vi "ABB Locked rotor report.vi"(10 "Report in":string) -> (2 "Report out":string, 3 "jpg  path":path)   [LabVIEW 2017]
uses:
  ABB global.vi
panel:
  out "Current Vs. Voltage":T1(graph)
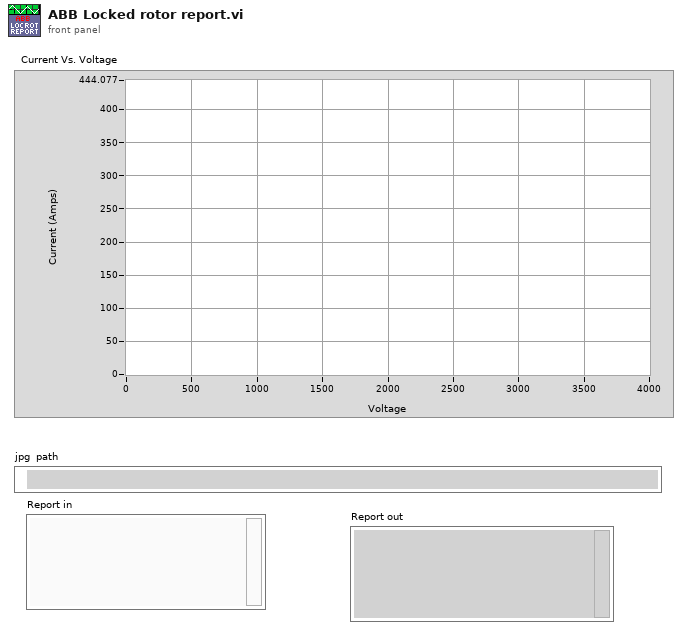
[diagram p1: front panel]
types:
  T1 = cluster{"No load test results":dbl[], "No load test results":dbl[]}
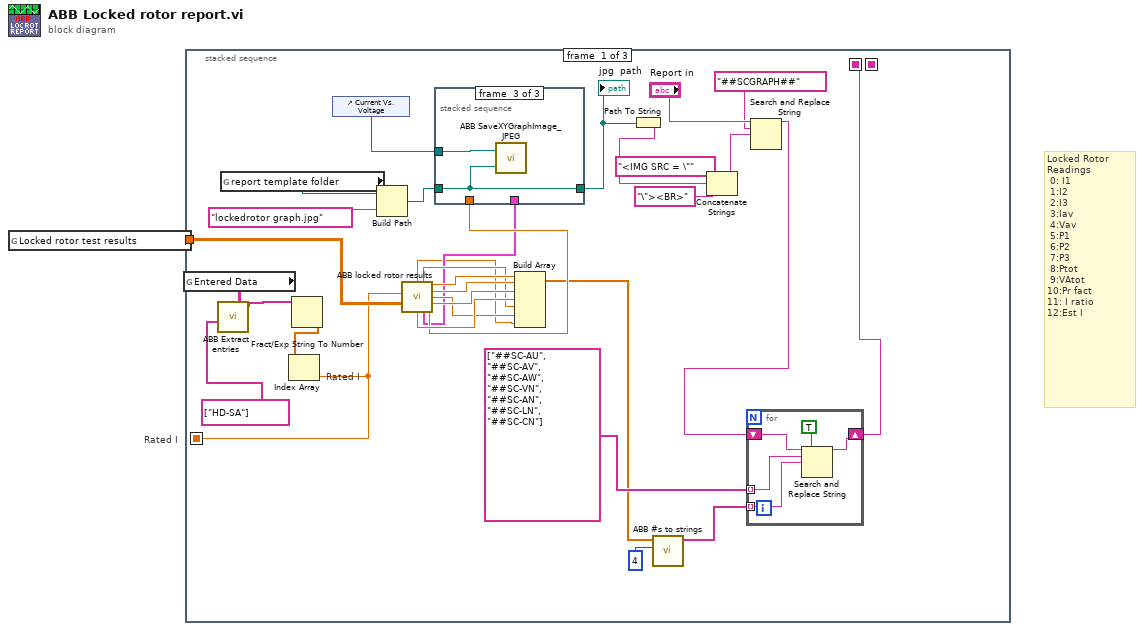
[diagram p0: block diagram]
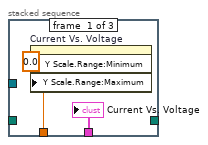
[diagram p2: hidden frame]
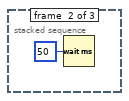
[diagram p3: hidden frame]
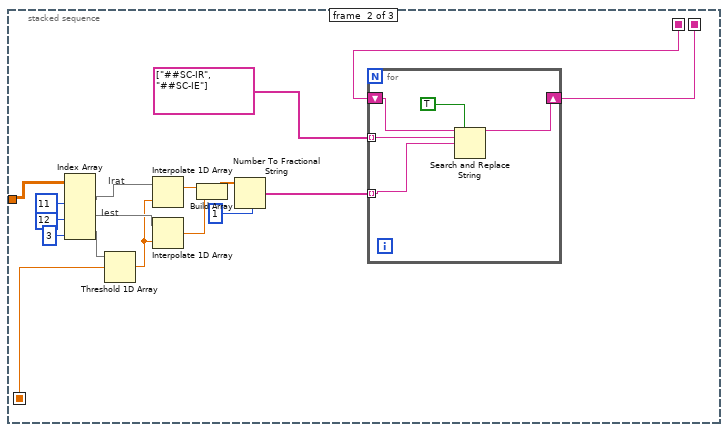
[diagram p4: hidden frame]
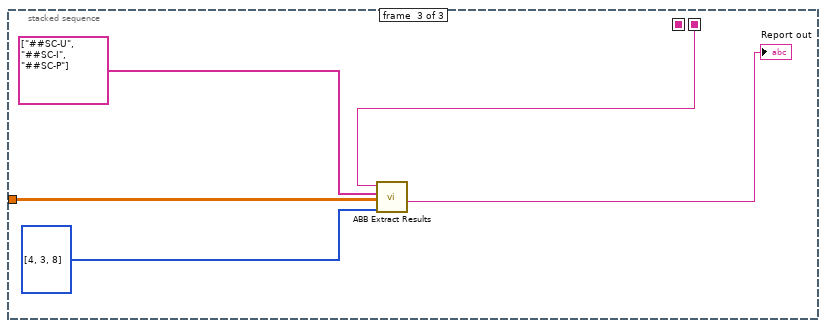
[diagram p5: hidden frame]
diagram:
  # "Rated I"
  # "Locked Rotor\nReadings\n 0: I1\n 1:I2\n 2:I3\n 3:Iav\n 4:Vav\n 5:P1\n 6:P2\n 7:P3\n 8:Ptot\n 9:VAtot\n10:Pr fact\n11: I ratio\n12:Est I"
  n1 = global read "ABB global.vi" "Locked rotor test results"() -> (w1:dbl[][])
  n2 = stacked-sequence {
    seq-local: [w20 _ _] -> [_ w49 _]
    seq-local: [_ w46 _] -> [_ _ w67]
    seq-local: [w3 _ _] -> [_ w45 _]
    tunnel: w1 -> [w15 w50 w71]
    frame #0 {
      # "Rated I"
      n3 = global read "ABB global.vi" "Entered Data"() -> (w23:string[][])
      n4 = call "ABB Extract entries.vi"("Entry IDs"=string[] ["HD-SA"], "Entry table in"=w23) -> ("Selected Entries"=w21:string[])  [unwired: 9 in]
      n5 = global read "ABB global.vi" "report template folder"() -> (w32:path)
      n6 = Fract/Exp String To Number(string=w21) -> (number=w14:dbl[])  [unwired: 3 in, 1 out]
      n7 = Index Array(array=w14) -> (element=w3:dbl)  [unwired: 1 in]
      n8 = control-ref of="Current Vs. Voltage"() -> (w33:refnum<vi>)
      n9 = Build Path(base path=w32, name or relative path="lockedrotor graph.jpg") -> (appended path=w28:path)
      n10 = call "ABB locked rotor results.vi"("Rated Current"=w3, "Locked rotor test results"=w15) -> ("PFr"=w4:dbl, "I AVr"=w9:dbl, "IUr"=w13:dbl, "IVr"=w12:dbl, "PWr"=w8:dbl, "IWr"=w11:dbl, "V AVr"=w10:dbl, "Graph"=w6:T1, "Max Value"=w7:dbl)  [unwired: 5 in]
      n11 = stacked-sequence {
        tunnel: w33 -> [_ _ w39]
        tunnel: w28 -> [_ _ w38]
        tunnel: w7 -> [w35 _ _]
        tunnel: w6 -> [w34 _ _]
        tunnel: [_ _ w38] -> w5
        frame #0 {
          n12 = property on="Current Vs. Voltage" class="XYGraph (strict)"("Y Scale.Range:Minimum"=0.0, "Y Scale.Range:Maximum"=w35) -> ()  [unwired: 2 in, 2 out]
          "Current Vs. Voltage" <- w34
        }
        frame #1 {
          n13 = Wait (ms)(milliseconds to wait=u32 50) -> ()  [unwired: 1 out]
        }
        frame #2 {
          n14 = call "ABB SaveXYGraphImage_JPEG.vi"("Path"=w38, "COntrolReference"=w39) -> ()  [unwired: 2 in]
        }
      }
      "jpg  path" <- w5
      n15 = Build Array(w13, w12, w11, w10, w9, w8, w4) -> (w2:dbl[])
      n16 = Path To String(path=w5) -> (string=w27:string)
      n17 = call "ABB #s to strings.vi"("Precision"=i16 4 ("precision (6)"), "Numbers in"=w2) -> ("Strings out"=w19:string[])  [unwired: 9 in]
      n18 = Concatenate Strings("<IMG SRC = \"", w27, "\"><BR>" ("string")) -> (w29:string)
      n19 = Search and Replace String(input string="Report in", search string="##SCGRAPH##", replace string=w29) -> (result string=w24:string)  [unwired: 5 in, 3 out]
      n20 = for {
        tunnel: string[] ["##SC-AU", "##SC-AV", "##SC-AW", "##SC-VN", "##SC-AN", "##SC-LN", "##SC-CN"] -> [w44] mode=indexing
        shift-right: [w42] -> w20
        shift-left: w24 -> [w43]
        tunnel: w19 -> [w41] mode=indexing
        n21 = Search and Replace String(replace all?=TRUE ("replace all? (F)"), input string=w43, search string=w44, replace string=w41) -> (result string=w42:string)  [unwired: 4 in, 3 out]
      }
    }
    frame #1 {
      # "Iest"
      # "Irat"
      n22 = Index Array(array=w50, index (col) #1=11 ("disabled index (col)"), index (col) #2=12 ("index (col)"), index (col) #3=3 ("index (col)")) -> (element #1=w57:dbl[], element #2=w56:dbl[], element #3=w58:dbl[])  [unwired: 3 in]
      n23 = Threshold 1D Array(2:w45, 3:w58) -> (0:w55:dbl)  [unwired: 1 in]
      n24 = Interpolate 1D Array(1:w55, 2:w57) -> (0:w53:dbl)
      n25 = Interpolate 1D Array(1:w55, 2:w56) -> (0:w52:dbl)
      n26 = Build Array(w53, w52) -> (w51:dbl[])
      n27 = Number To Fractional String(number=w51, precision (6)=i16 1) -> (F-format string=w47:string[])  [unwired: 2 in]
      n28 = for {
        shift-right: [w63] -> w46
        shift-left: w49 -> [w65]
        tunnel: string[] ["##SC-IR", "##SC-IE"] -> [w66] mode=indexing
        tunnel: w47 -> [w62] mode=indexing
        n29 = Search and Replace String(replace all?=TRUE ("replace all? (F)"), input string=w65, search string=w66, replace string=w62) -> (result string=w63:string)  [unwired: 4 in, 3 out]
      }
    }
    frame #2 {
      n30 = call "ABB Extract Results.vi"("Column#"=i32[] [4, 3, 8], "test results"=w71, "ID group"=string[] ["##SC-U", "##SC-I", "##SC-P"], "Report in"=w67) -> ("Report Out"=→"Report out":string)  [unwired: 7 in]
    }
  }
